vi "Standard Controls Module.vi"(0 "FPGA VI Reference In":refnum<k20>, 1 "Control Type":bool, 5 "Command":T5(ring), 7 "Servo Motors Control":T3={"Base"=500, "Elbow"=500, "Claw"=500, "Shoulder"=500} {"Shoulder" min=500 max=2250 scale=0.0..200.0; "Claw" min=500 max=2250 scale=145.0..175.0; "Elbow" min=500 max=2250 scale=0.0..200.0; "Base" min=500 max=2250 scale=0.0..200.0}, 9 "Obstacle Data":T2, 11 "Error In":errorcluster, 12 "Speed":T1, 13 "Buttons Control":T4, 14 "Arm":enum32{"meArm", "uArm"}(ring)) -> (3 "Output":string, 4 "FPGA VI Reference Out":refnum<k20>, 15 "Error Out":errorcluster)   [LabVIEW 2015]
uses:
  Utilities/Error.ctl
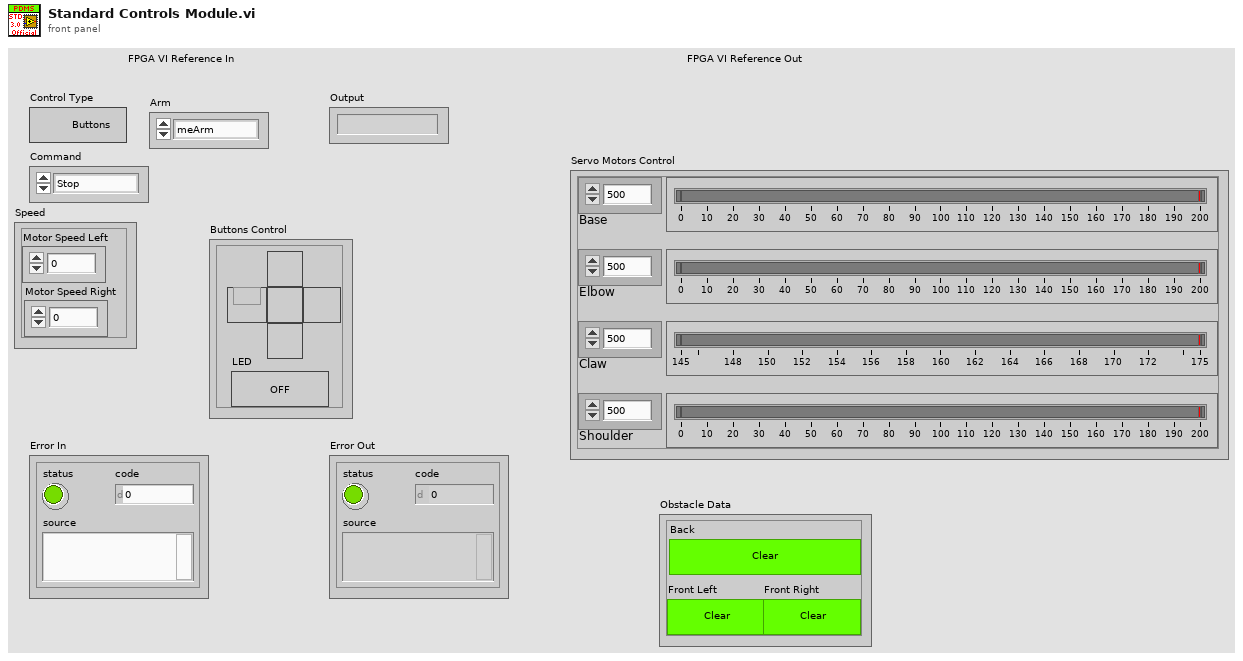
[diagram p1: front panel]
types:
  T1 = cluster{"Motor Speed Left":i16, "Motor Speed Right":i16}
  T2 = cluster{"Back":bool, "Front Left":bool, "Front Right":bool}
  T3 = cluster{"Base":u16, "Elbow":u16, "Claw":u16, "Shoulder":u16}
  T4 = cluster{"Front":bool, "Right":bool, "Back":bool, "Left":bool, "Stop":bool, "LED":bool}
  T5 = enum16{"Stop", "LED", "Front", "Back", "Left", "Right"}
  T6 = cluster{"LED 1":enum16{"Brightness", "Bool"}, "BOOL":bool, "Brightness":u32}
  T7 = typedef "Error.ctl" = enum16{"No Error", "Custom", "Standard", "GPS Signal", "YH Left", "YL Right", "XL Back", "XH Front"}
  T8 = cluster{"I 1":bool, "I 2":bool, "I 3":bool, "I 4":bool}
  T9 = typedef "DIR GAME.ctl" = enum16{"Stop", "Front", "FR", "Right", "BR", "Back", "BL", "Left", "FL"}
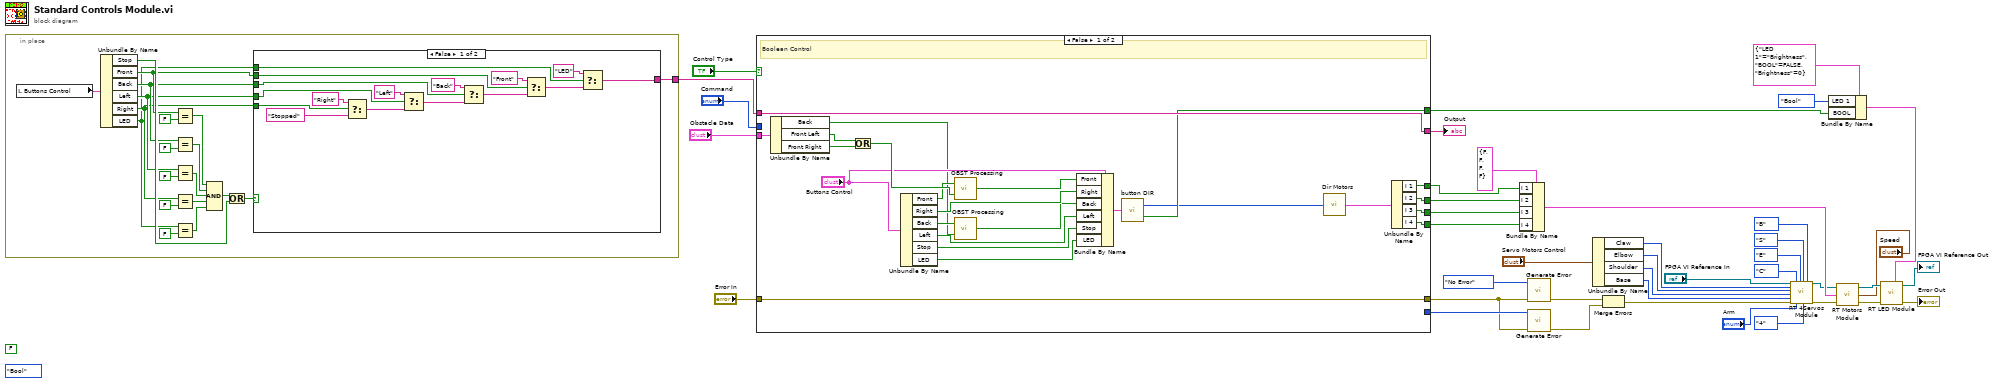
[diagram p0: block diagram]
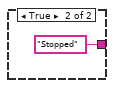
[diagram p2: hidden frame]
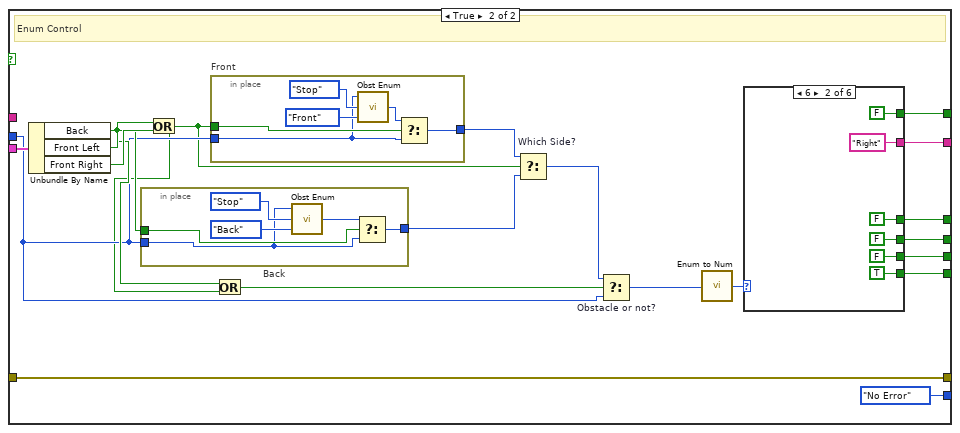
[diagram p3: hidden frame]
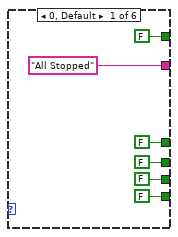
[diagram p4: hidden frame]
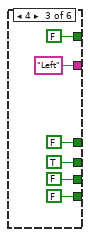
[diagram p5: hidden frame]
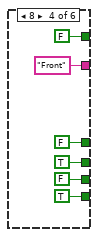
[diagram p6: hidden frame]
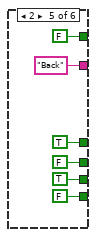
[diagram p7: hidden frame]
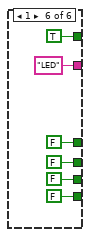
[diagram p8: hidden frame]
diagram:
  (unwired) FALSE ("Stop Button")
  (unwired) enum16{"Brightness", "Bool"}."Bool" ("LED")
  n1 = in-place {
    in-place-border: [w42] -> w10
    n2 = local read "Buttons Control"() -> (w50:T4)
    n3 = Unbundle By Name(w50) -> ("Stop"=w49:bool, "Front"=w47:bool, "Back"=w46:bool, "Left"=w45:bool, "Right"=w44:bool, "LED"=w43:bool)
    n4 = Equal?(x=w47, y=FALSE ("Control Type")) -> (x = y?=w56:bool)
    n5 = Equal?(x=w46, y=FALSE ("Control Type")) -> (x = y?=w55:bool)
    n6 = Equal?(x=w45, y=FALSE ("Control Type")) -> (x = y?=w54:bool)
    n7 = Equal?(x=w44, y=FALSE ("Control Type")) -> (x = y?=w53:bool)
    n8 = Equal?(x=w43, y=FALSE ("Control Type")) -> (x = y?=w52:bool)
    n9 = Compound Arithmetic op=AND(w56, w55, w54, w53, w52) -> (w51:bool)
    n10 = Or(x=w51, y=w49) -> (x .or. y?=w48:bool)
    n11 = case shown="False" w48 {
      tunnel: [w64 "Stopped"] -> w42
      tunnel: w47 -> [w77 _]
      tunnel: w46 -> [w75 _]
      tunnel: w45 -> [w73 _]
      tunnel: w44 -> [w71 _]
      tunnel: w43 -> [w62 _]
      frame False {
        n12 = Select(t="Right", s=w71, f="Stopped") -> (s? t:f=w72:string)
        n13 = Select(t="Left", s=w73, f=w72) -> (s? t:f=w74:string)
        n14 = Select(t="Back", s=w75, f=w74) -> (s? t:f=w76:string)
        n15 = Select(t="Front", s=w77, f=w76) -> (s? t:f=w65:string)
        n16 = Select(t="LED", s=w62, f=w65) -> (s? t:f=w64:string)
      }
      frame True {
      }
    }
  }
  n17 = case shown="False" "Control Type" {
    tunnel: "Command" -> [_ w108]
    tunnel: "Error In" -> [w102 w122]
    tunnel: [w102 w122] -> w12
    tunnel: [_ Error."No Error" ("Error??")] -> w26
    tunnel: [w82 w119] -> w21
    tunnel: [w84 w118] -> w20
    tunnel: [w85 w117] -> w19
    tunnel: [w83 w116] -> w18
    tunnel: [w95 w120] -> w7
    tunnel: [w98 w115] -> w16
    tunnel: "Obstacle Data" -> [w99 w113]
    tunnel: w10 -> [w98 _]
    frame False {
      # "Boolean Control"
      n18 = Unbundle By Name(w99) -> ("Back"=w79:bool, "Front Left"=w100:bool, "Front Right"=w101:bool)
      n19 = Or(x=w100, y=w101) -> (x .or. y?=w97:bool)
      n20 = Unbundle By Name("Buttons Control") -> ("Front"=w96:bool, "Right"=w90:bool, "Back"=w80:bool, "Left"=w89:bool, "Stop"=w87:bool, "LED"=w86:bool)
      n21 = call "OBST Processing.vi"("OBST"=w97, "Line"=w96) -> ("O/P"=w91:bool)
      n22 = call "OBST Processing.vi"("OBST"=w79, "Line"=w80) -> ("O/P"=w88:bool)
      n23 = Bundle By Name(cluster="Buttons Control", "Front"=w91, "Right"=w90, "Back"=w88, "Left"=w89, "Stop"=w87, "LED"=w86) -> (w92:T4)
      n24 = call "button DIR.vi"("Buttons Control"=w92) -> ("Direction 2"=w94:T9, "LED"=w95:bool)
      n25 = call "Dir Motors.vi"("Direction 2"=w94) -> ("A"=w81:T8)
      n26 = Unbundle By Name(w81) -> ("I 1"=w85:bool, "I 2"=w84:bool, "I 3"=w83:bool, "I 4"=w82:bool)
    }
    frame True {
      # "Enum Control"
      n27 = Unbundle By Name(w113) -> ("Back"=w110:bool, "Front Left"=w112:bool, "Front Right"=w111:bool)
      n28 = in-place "Back" {
        in-place-border: w110 -> [w128]
        in-place-border: w108 -> [w124]
        in-place-border: [w123] -> w105
        n29 = call "Obst Enum.vi"("Obstacle Side"=T5."Back", "If Obstacle"=T5."Stop", "Command"=w124) -> ("Out"=w126:T5)
        n30 = Select(t=w126, s=w128, f=w124) -> (s? t:f=w123:T5)
      }
      n31 = Or(x=w112, y=w111) -> (x .or. y?=w107:bool)
      n32 = in-place "Front" {
        in-place-border: w107 -> [w134]
        in-place-border: w108 -> [w130]
        in-place-border: [w129] -> w106
        n33 = call "Obst Enum.vi"("Obstacle Side"=T5."Front", "If Obstacle"=T5."Stop", "Command"=w130) -> ("Out"=w131:T5)
        n34 = Select(t=w131, s=w134, f=w130) -> (s? t:f=w129:T5)
      }
      n35 = Or(x=w110, y=w107) -> (x .or. y?=w109:bool)
      n36 = Select "Which Side?"(t=w106, s=w107, f=w105) -> (s? t:f=w104:T5)
      n37 = Select "Obstacle or not?"(t=w104, s=w109, f=w108) -> (s? t:f=w103:T5)
      n38 = call "Enum to Num.vi"("Command"=w103) -> ("Std Command"=w121:i32)
      n39 = case shown="6" w121 {
        tunnel: [FALSE TRUE FALSE TRUE FALSE FALSE] -> w119
        tunnel: [FALSE ("Boolean") FALSE ("Boolean") FALSE ("Boolean") FALSE TRUE FALSE] -> w117
        tunnel: [FALSE ("Boolean") FALSE TRUE TRUE FALSE FALSE] -> w118
        tunnel: [FALSE FALSE FALSE FALSE TRUE FALSE] -> w116
        tunnel: [FALSE FALSE FALSE FALSE FALSE TRUE] -> w120
        tunnel: ["All Stopped" "Right" "Left" "Front" "Back" "LED"] -> w115
        frame 0, Default {
        }
        frame 6 {
        }
        frame 4 {
        }
        frame 8 {
        }
        frame 2 {
        }
        frame 1 {
        }
      }
    }
  }
  "Output" <- w16
  n40 = Bundle By Name(cluster=T8 {"I 1"=FALSE, "I 2"=FALSE, "I 3"=FALSE, "I 4"=FALSE} ("A"), "I 1"=w19, "I 2"=w20, "I 3"=w18, "I 4"=w21) -> (w22:T8)
  n41 = call "Generate Error.vi"("Error In"=w12, "Enum"=Error."No Error") -> ("Error Out"=w24:errorcluster)  [unwired: 9 in]
  n42 = call "Generate Error.vi"("Error In"=w12, "Enum"=w26) -> ("Error Out"=w25:errorcluster)  [unwired: 9 in]
  n43 = Unbundle By Name("Servo Motors Control") -> ("Claw"=w41:u16, "Elbow"=w40:u16, "Shoulder"=w39:u16, "Base"=w38:u16)
  n44 = Merge Errors(w24, w25) -> (w15:errorcluster)
  n45 = call "RT 4Servos Module.vi"("FPGA VI Reference In"="FPGA VI Reference In", "Angle 1"=w41, "Angle 2"=w40, "Angle 3"=w39, "Angle 4"=w38, "Error In"=w15, "Motor 1"=enum16{"B", "S", "E", "C"}."C", "Arm"="Arm", "Motor 2"=enum16{"B", "S", "E", "C"}."E", "Motor 3"=enum16{"B", "S", "E", "C"}."S", "No. of Motors"=enum16{"1", "2", "3", "4"}."4", "Motor 4"=enum16{"B", "S", "E", "C"}."B") -> ("FPGA VI Reference Out"=w2:refnum<k20>, "Error Out"=w32:errorcluster)  [unwired: 6 in]
  n46 = Bundle By Name(cluster=T6 {"LED 1"=enum."Brightness", "BOOL"=FALSE, "Brightness"=0} ("LED 1"), "LED 1"=enum16{"Brightness", "Bool"}."Bool", "BOOL"=w7) -> (w6:T6)
  n47 = call "RT Motors Module.vi"("Speed"="Speed", "Error In"=w32, "All"=w22, "FPGA VI Reference In"=w2) -> ("Error Out"=w31:errorcluster, "FPGA VI Reference Out"=w23:refnum<k20>)
  n48 = call "RT LED Module.vi"("LED 1"=w6, "error in"=w31, "FPGA VI Reference In"=w23) -> ("error out"=→"Error Out":errorcluster, "FPGA VI Reference Out"=→"FPGA VI Reference Out":refnum<k20>)  [unwired: 7 in]
